vi "Configure Reference Level.vi"(6 "Reference Type to Configure (0: Pulse Duration Reference Levels)":i32(ring) items=["Pulse Duration Reference Levels", "Transition Duration and Occurrences Reference Levels"], 7 "Occurrences Reference Levels (90)":dbl=90.0, 8 "error in (no error)":errorcluster, 9 "Transition Duration Reference Levels (10)":dbl=10.0, 10 "Pulse Duration Reference Levels (50)":dbl=50.0, 11 "VISA resource name":refnum<visa-resource-name>) -> (0 "error out":errorcluster, 3 "VISA resource name out":refnum<visa-resource-name>)   [LabVIEW 2018, in "Agilent U2000 Series.lvlib"]
doc: "Defines the reference levels.\n\nNote:\nFor U2040 X-Series, this VI is applicable for U2042XA/U2044XA/U2049XA models."
uses:
  Agilent U2000 Series.lvlib
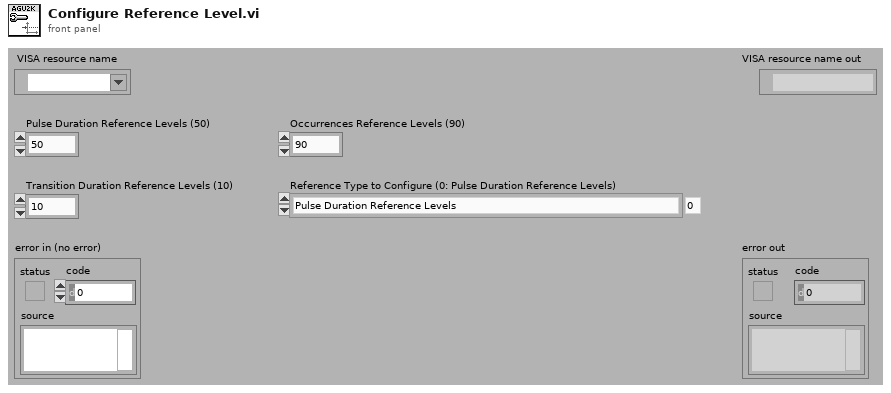
[diagram p1: front panel]
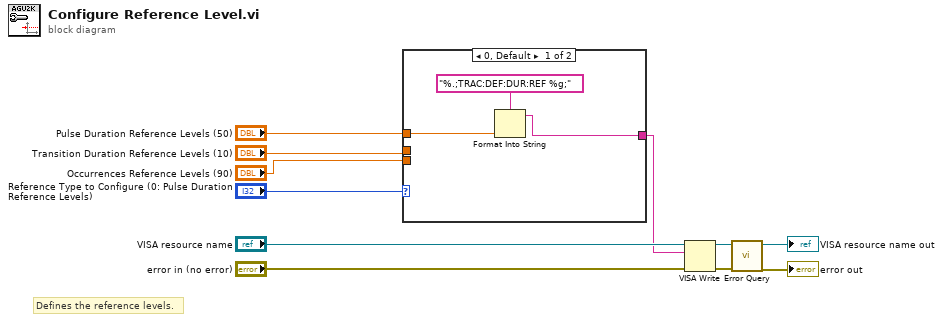
[diagram p0: block diagram]
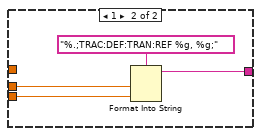
[diagram p2: hidden frame]
diagram:
  # "Defines the reference levels."
  n1 = case shown="0, Default" "Reference Type to Configure (0: Pulse Duration Reference Levels)" {
    tunnel: "Pulse Duration Reference Levels (50)" -> [w13 _]
    tunnel: [w12 w15] -> w3
    tunnel: "Transition Duration Reference Levels (10)" -> [_ w17]
    tunnel: "Occurrences Reference Levels (90)" -> [_ w16]
    frame 0, Default {
      n2 = Format Into String(format string="%.;TRAC:DEF:DUR:REF %g;", w13) -> (resulting string=w12:string)  [unwired: 2 in, 1 out]
    }
    frame 1 {
      n3 = Format Into String(format string="%.;TRAC:DEF:TRAN:REF %g, %g;", w17, w16) -> (resulting string=w15:string)  [unwired: 2 in, 1 out]
    }
  }
  n4 = VISA Write(VISA resource name="VISA resource name", write buffer=w3, error in (no error)="error in (no error)") -> (VISA resource name out=w9:refnum<visa-resource-name>, error out=w8:errorcluster)  [unwired: 1 out]
  n5 = call "Error Query.vi"("error in (no error)"=w8, "VISA resource name"=w9) -> ("error out"=→"error out":errorcluster, "VISA resource name out"=→"VISA resource name out":refnum<visa-resource-name>)  [unwired: 8 out]
